vi "sort_even.vi"() -> ()   [LabVIEW 2020]
panel:
  out "Array":i32[](array[numeric])
  # "Sort Even Numbers"
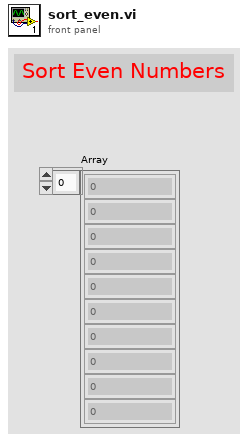
[diagram p1: front panel]
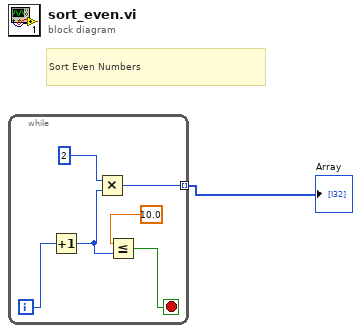
[diagram p0: block diagram]
diagram:
  # "Sort Even Numbers"
  n1 = while {
    tunnel: [w2] -> w1 mode=indexing
    i -> [w4]
    stop <- w3 stop-if-true
    n2 = Increment(x=w4) -> (x+1=w6:i32)
    n3 = Multiply(x=2, y=w6) -> (x*y=w2:i32)
    n4 = Less Or Equal?(x=10.0, y=w6) -> (x <= y?=w3:bool)
  }
  "Array" <- w1
